vi "User Interface References.vi"(7 "Set or Get Value":enum16{"Set", "Get"}(ring), 8 "error in":errorcluster, 11 "Display State In":T1={"Numeric"=0.0, "Array of Button References"=[], "Space Between Menu Buttons"=0, "Number of Menu Buttons"=0, "Array of Button Names"=[], "Most Recent Vertical Position"=0, "This VI"=refnum, "Current Action"=enum."Not Moving", "Most Recent Distance Traveled"=0, "Method"=enum."Move Up", "Data In"=0}) -> (0 "error out":errorcluster, 3 "Display State Out":T1={"Numeric"=0.0, "Array of Button References"=[], "Space Between Menu Buttons"=0, "Number of Menu Buttons"=0, "Array of Button Names"=[], "Most Recent Vertical Position"=0, "This VI"=refnum, "Current Action"=enum."Not Moving", "Most Recent Distance Traveled"=0, "Method"=enum."Move Up", "Data In"=0} caption="State")   [LabVIEW 2011, in "Sliding Menu Library.lvlib" / "Sliding Menu XControl.xctl"]
uses:
  Sliding Menu xControl/Sliding Menu XControl.xctl
  Sliding Menu xControl/Sliding Menu State.ctl
  Menu Button Library/Menu Button xControl/Menu Button xControl.xctl
  Sliding Menu Type Definitions/Current User Action.ctl
  Sliding Menu xControl/Sliding Menu Methods.ctl
  Sliding Menu xControl/Sliding Menu Data.ctl
  Sliding Menu Library.lvlib
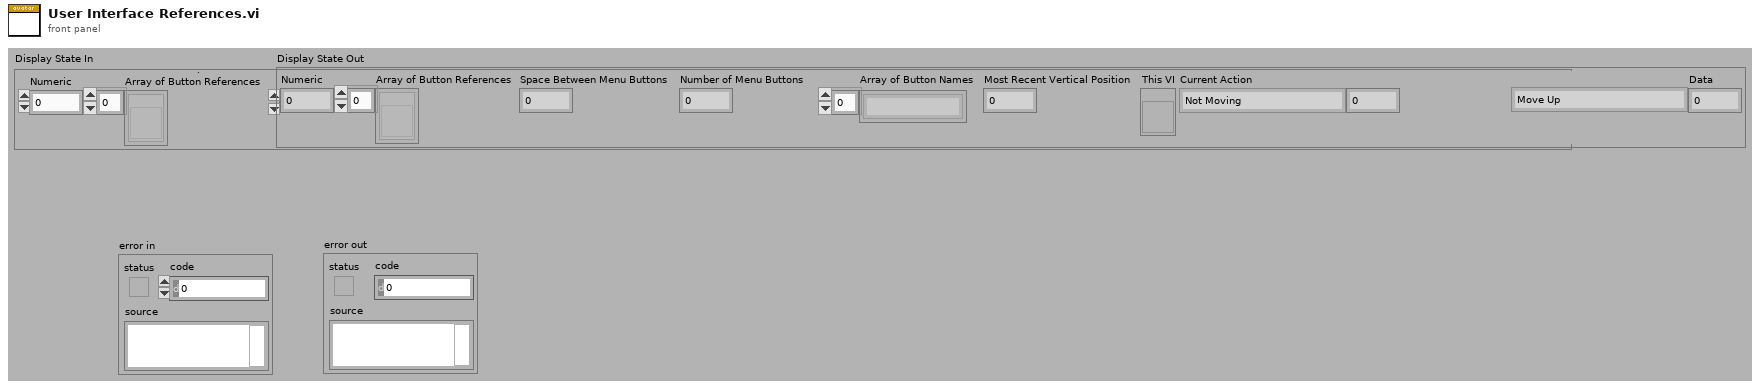
[diagram p1: front panel]
types:
  T1 = typedef "Sliding Menu Library.lvlib/Sliding Menu XControl.xctl/Sliding Menu State.ctl" = cluster{"Numeric":dbl, "Array of Button References":refnum<vi>[], "Space Between Menu Buttons":i32, "Number of Menu Buttons":i32, "Array of Button Names":string[], "Most Recent Vertical Position":i32, "This VI":refnum<vi>, "Current Action":T2, "Most Recent Distance Traveled":i32, "Method":T3, "Data In":T4}
  T2 = typedef "Sliding Menu Library.lvlib/Current User Action.ctl" = enum16{"Not Moving", "Mouse Down", "Mouse Up No Dragging", "Bounce Up Needed", "Bounce Down Needed", "Dragging", "Easing"}
  T3 = typedef "Sliding Menu Methods.ctl" = enum16{"Resize", "Move Up", "Move Down", "Move to 0"}
  T4 = typedef "Sliding Menu Library.lvlib/Sliding Menu XControl.xctl/Sliding Menu Data.ctl" = i32
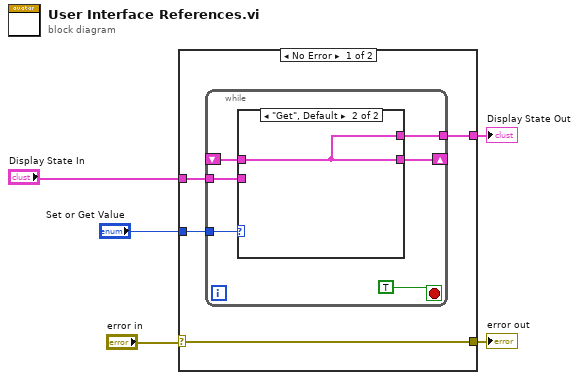
[diagram p0: block diagram]
diagram:
  n1 = case shown="No Error" "error in" {
    selector: "error in" -> [w7 w18]
    tunnel: "Set or Get Value" -> [w9 _]
    tunnel: "Display State In" -> [w8 _]
    tunnel: [w7 w18] -> w3
    tunnel: [w6 _] -> w1
    frame No Error {
      n2 = while {
        tunnel: w8 -> [w14]
        shift-right: [w11] -> _
        shift-left: _ -> [w13]
        tunnel: w9 -> [w12]
        tunnel: [w10] -> w6
        stop <- TRUE stop-if-true
        n3 = case shown="\"Get\", Default" w12 {
          tunnel: w14 -> [w16 _]
          tunnel: [w16 w17] -> w11
          tunnel: w13 -> [_ w17]
          tunnel: [w16 w17] -> w10
          frame "Set" {
          }
          frame "Get", Default {
          }
        }
      }
    }
    frame Error {
    }
  }
  "error out" <- w3
  "Display State Out" <- w1
